vi "Main.vi"() -> ()   [LabVIEW 2017]
uses:
  <vilib>/Platform/TimedLoop/XDataNode/timing_clust.ctl
  <vilib>/Platform/TimedLoop/XDataNode/nitl_modes.ctl
  <vilib>/Platform/TimedLoop/XDataNode/wakeup.ctl
  <vilib>/Analysis/Matrix/Datatypes/RealMatrix.ctl
  <vilib>/Analysis/baseanly.llb/A x Vector.vi
  <vilib>/Analysis/baseanly.llb/Real A x B.vi
  <vilib>/Analysis/_algsub.llb/Real Vector Norm.vi
  <vilib>/Analysis/baseanly.llb/Outer Product.vi
  <vilib>/Analysis/baseanly.llb/Real Outer Product.vi
  <vilib>/robotics/Kinematics/Create Lie Group Matrix.vi
  <vilib>/Analysis/7linalg.llb/Create Special Matrix.vi
  <vilib>/Analysis/7linalg.llb/Create Special Real Matrix.vi
  <vilib>/Analysis/Matrix/Numeric/Multiply/Multiply.vi
  <vilib>/Analysis/Matrix/Numeric/Multiply/Multiply - RM,R.vi
  <vilib>/Analysis/Matrix/Numeric/Multiply/Multiply - R,RM.vi
  <vilib>/Analysis/Matrix/Numeric/Add/Add.vi
  <vilib>/Analysis/Matrix/Numeric/Add/Add - RM,RM.vi
  <vilib>/platform/TimedLoop/XDataNode/XDataNode.xnode
  <vilib>/robotics/Kinematics/NI_Kinematics.lvlib
  <vilib>/Analysis/NI_AALBase.lvlib
  <vilib>/Platform/TimedLoop/XDataNode/XDNodeRunTimeDep.lvlib
  <vilib>/Native 3D Graph/xcontrol/3DPC_SurfacePlot.xctl
  <vilib>/Analysis/Matrix/NI_Matrix.lvlib
  <vilib>/Analysis/NI_AALPro.lvlib
  <vilib>/Native 3D Graph/classes/Base Datatype.lvclass
panel:
  out "W-L":dbl=9.959
  out "break":bool=TRUE
  out "state":dbl[](array[numeric])=[1.0, 0.5, 0.5]
  in  "rom":dbl=0.5
  out "target":dbl[](array[numeric])=[inf, inf, inf] format="%#_15g"
  out "chromosome":dbl[](array[numeric])=[0.20251449555250356, 0.8674619116743827, 0.35840498316248204, 0.9462828018798735, 0.6979927649497852, 0.5023536487970717]
  in  "inertia":dbl=1.0
  out "torque":dbl[](array[numeric])
  in  "radius":dbl=1.0
  in  "damping":dbl=0.5
  out "beta2":dbl=0.7460127831658564
  out "v30":dbl[](array[numeric])=[0.5877852522924729, -0.33935797363675174, -0.7344008870614411]
  out "v10":dbl[](array[numeric])=[0.0, 0.6787159472735029, -0.7344008870614411]
  out "v20":dbl[](array[numeric])=[-0.5877852522924731, -0.3393579736367513, -0.7344008870614411]
  out "dt":dbl=0.001
  in  "period":i64=1
  out "v2":dbl[](array[numeric])=[-0.5877852522924731, -0.3393579736367513, -0.7344008870614411]
  out "v1":dbl[](array[numeric])=[0.0, 0.6787159472735029, -0.7344008870614411]
  out "v3":dbl[](array[numeric])=[0.5877852522924729, -0.33935797363675174, -0.7344008870614411]
  out "theta":dbl[](array[numeric]) format="%#_15g"
  in  "stop":bool
  out "beta1":dbl=0.9553166181245093
  out "gamma2":dbl=1.2566370614359172
  out "gamma1":dbl=1.5707963267948966
  out "alpha2":dbl=1.5707963267948966
  out "alpha1":dbl=1.5707963267948966
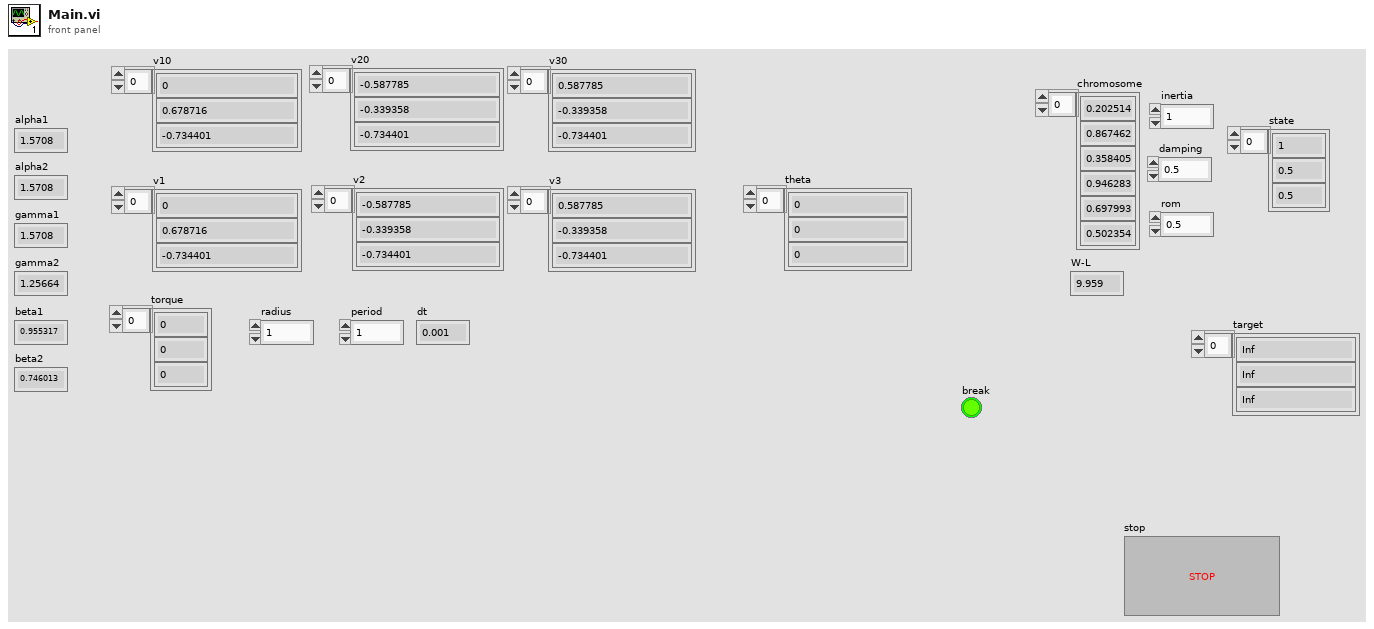
[diagram p1: front panel]
types:
  T1 = typedef "XDNodeRunTimeDep.lvlib/timing_clust.ctl" = cluster{"Expected End [f-1]":u64, "Actual End [f-1]":u64, "Finished Late? [f-1]":bool, "Expected End [i-1]":u64, "Actual End [i-1]":u64, "Finished Late? [i-1]":bool, "Expected Start [i]":u64, "Actual Start [i]":u64, "Expected Start [f]":u64, "Actual Start [f]":u64, "Source Name":string, "Structure Name":string, "Period":i64, "Deadline":i64, "Offset":i64, "Start":i64, "Priority":i32, "Timeout":i32, "Mode":T2, "Wakeup Reason":T3, "Error":errorcluster, "Source Type":string, "Secondary Source Type":string, "Global End Time":u64, "Global Start Time":u64, "Frame Duration":u64, "Iteration Duration":u64, "Assigned CPU":i32, "I/O Scan Engine Mode":u32}
  T2 = typedef "XDNodeRunTimeDep.lvlib/nitl_modes.ctl" = enum32{"No Change", "Process missed periods, maintain original phase", "Discard missed periods, maintain original phase", "Process missed periods, ignore original phase", "Discard missed periods, ignore original phase"}
  T3 = typedef "XDNodeRunTimeDep.lvlib/wakeup.ctl" = enum32{"Normal", "Aborted", "Asynchronous wakeup", "Timing source error", "Timed loop error", "Timeout"}
  T4 = typedef "NI_Matrix.lvlib/RealMatrix.ctl" = dbl[][]
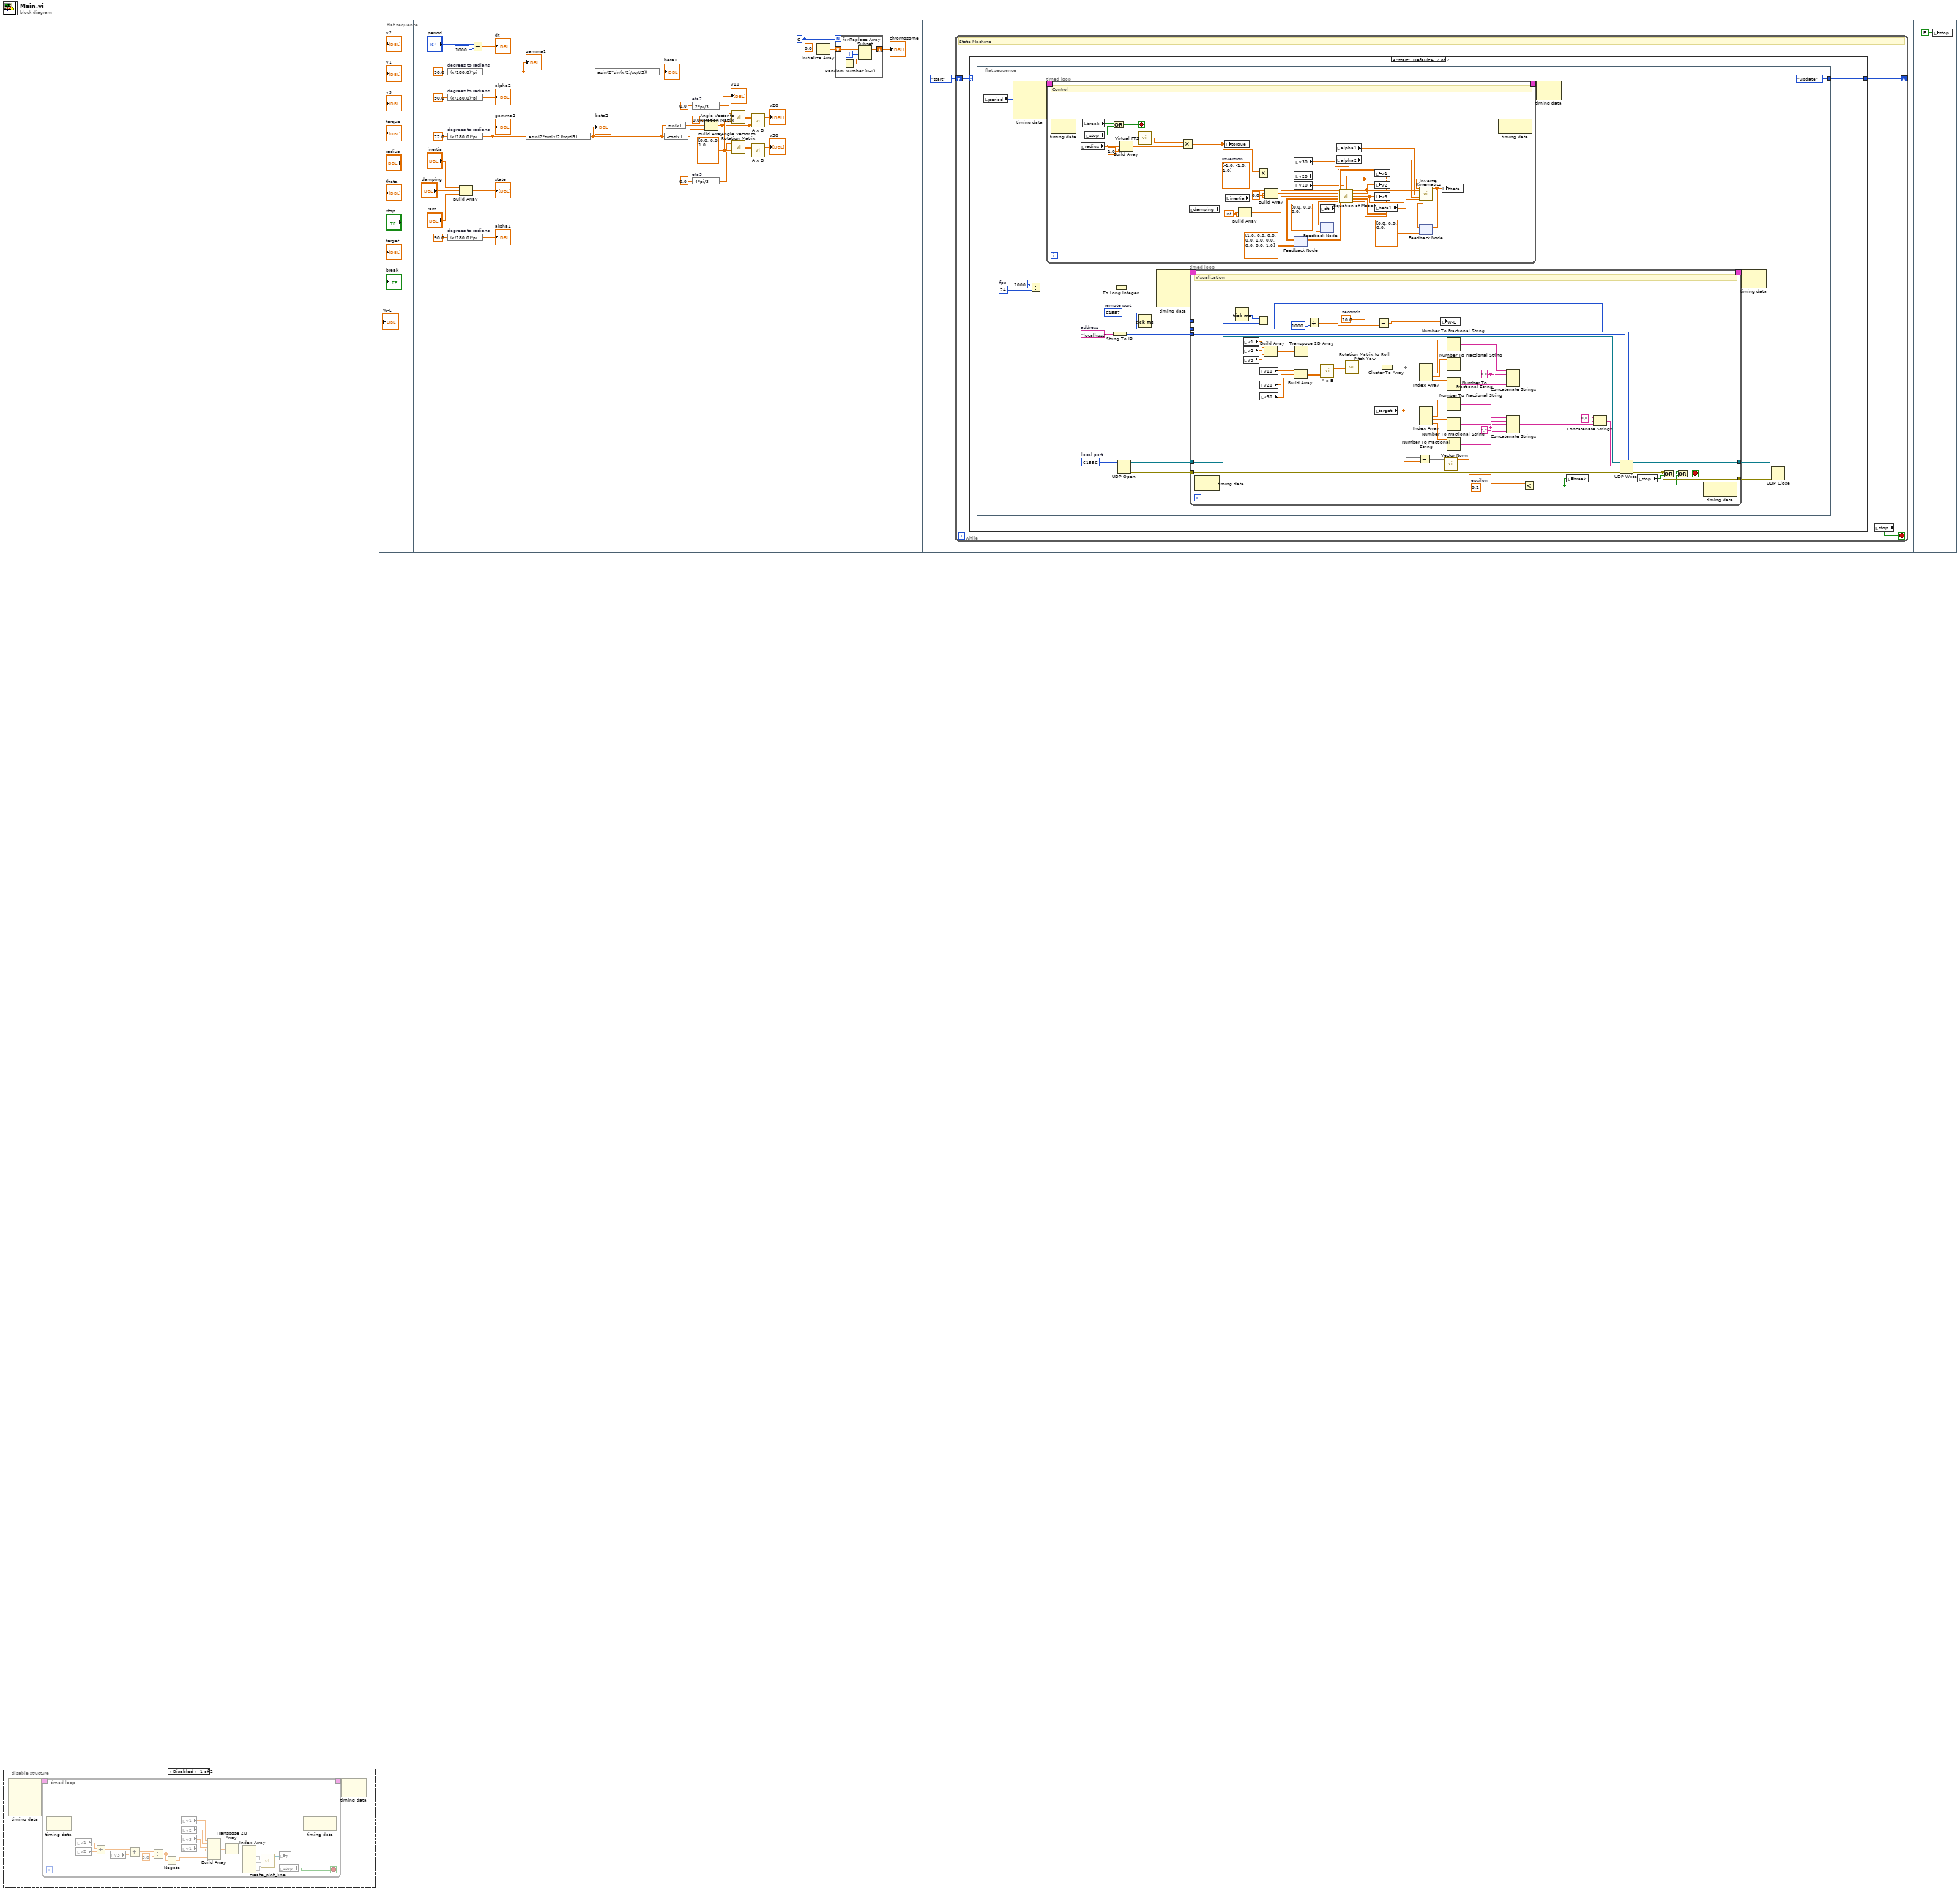
[diagram p0: block diagram]
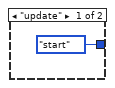
[diagram p3: hidden frame]
diagram:
  n1 = disable-structure shown="Disabled" {
    frame Disabled {
      n2 = node-c288() -> (w2:T1)  [unwired: 4 in]
      n3 = timed-loop {
        timing: w2 -> [_]
        timing-out: [_] -> w1
        stop <- w3 stop-if-true
        n4 = node-c288() -> ()  [unwired: 1 in, 1 out]
        n5 = local read "v1"() -> (w12:dbl[])
        n6 = local read "v2"() -> (w11:dbl[])
        n7 = Add(x=w12, y=w11) -> (x+y=w10:dbl[])
        n8 = local read "v3"() -> (w9:dbl[])
        n9 = Add(x=w10, y=w9) -> (x+y=w8:dbl[])
        n10 = Divide(x=w8, y=3.0) -> (x/y=w6:dbl[])
        n11 = Negate(x=w6) -> (-x=w5:dbl[])
        n12 = local read "v1"() -> (w20:dbl[])
        n13 = local read "v2"() -> (w19:dbl[])
        n14 = local read "v3"() -> (w18:dbl[])
        n15 = local read "v1"() -> (w17:dbl[])
        n16 = Build Array(w20, w19, w18, w17, w6, w5) -> (w16:dbl[][])
        n17 = Transpose 2D Array(2D array=w16) -> (transposed array=w15:dbl[][])
        n18 = Index Array(array=w15) -> (element #1=w14:dbl[], element #2=w13:dbl[], element #3=w4:dbl[])  [unwired: 6 in]
        n19 = call <vilib>:"create_plot_line.vi"("z vector"=w4, "y vector"=w13, "x vector"=w14) -> ("plots out"=w21:refnum<class "Base Datatype.lvclass">[])  [unwired: 2 in, 6 out]
        n20 = local write item#-1(w21) -> ()
        n21 = local read "stop"() -> (w3:bool)
        n22 = node-c288() -> ()  [unwired: 1 in, 1 out]
      }
      n23 = node-c288(w1) -> ()  [unwired: 1 out]
    }
    frame Enabled {
    }
  }
  n24 = flat-sequence {
    frame #0 {
    }
    frame #1 {
      w52 = dbl[] [0.0, 0.0, 1.0] ("vector")
      # "Kinematics Variables"
      n25 = expression code="(x/180.0)*pi" "degrees to radians"(90.0 ("gamma1")) -> (w36:dbl)
      "gamma1" <- w36
      n26 = expression code="(x/180.0)*pi" "degrees to radians"(90.0 ("alpha2")) -> (→"alpha2":dbl)
      n27 = expression code="(x/180.0)*pi" "degrees to radians"(72.0 ("gamma2")) -> (w34:dbl)
      "gamma2" <- w34
      n28 = expression code="(x/180.0)*pi" "degrees to radians"(90.0 ("alpha1")) -> (→"alpha1":dbl)
      n29 = Build Array("inertia", "damping", "rom") -> (→"state":dbl[])
      n30 = Divide(x="period", y=i64 1000) -> (x/y=→"dt":dbl)
      n31 = expression code="asin(2*sin(x/2)/sqrt(3))"(w34) -> (w30:dbl)
      "beta2" <- w30
      n32 = expression code="asin(2*sin(x/2)/sqrt(3))"(w36) -> (→"beta1":dbl)
      n33 = expression code="-cos(x)"(w30) -> (w53:dbl)
      n34 = expression code="sin(x)"(w30) -> (w54:dbl)
      n35 = expression code="2*pi/3" "eta2"(0.0) -> (w51:dbl)
      n36 = expression code="4*pi/3" "eta3"(0.0) -> (w50:dbl)
      n37 = Build Array(0.0 ("element"), w54, w53) -> (w45:dbl[])
      "v10" <- w45
      n38 = call <vilib>:"Angle Vector to Rotation Matrix.vi"("vector"=w52, "angle"=w51) -> ("rotation matrix"=w49:T4)
      n39 = call <vilib>:"Angle Vector to Rotation Matrix.vi"("vector"=w52, "angle"=w50) -> ("rotation matrix"=w48:T4)
      n40 = call-poly <vilib>:"A x B.vi"("Vector"=w45, "A"=w49) -> ("A x Vector"=→"v20":dbl[])  [unwired: 1 out]
      n41 = call-poly <vilib>:"A x B.vi"("Vector"=w45, "A"=w48) -> ("A x Vector"=→"v30":dbl[])  [unwired: 1 out]
    }
    frame #2 {
      w57 = 6
      n42 = Initialize Array(0.0 ("element"), w57) -> (w59:dbl[])
      n43 = for {
        N: w57 -> [_]
        shift-right: [w60] -> w56
        shift-left: w59 -> [w63]
        i -> [w62]
        n44 = Random Number (0-1)() -> (number: 0 to 1=w61:dbl)
        n45 = Replace Array Subset(array=w63, new element=w61, index=w62) -> (w60:dbl[])
      }
      "chromosome" <- w56
    }
    frame #3 {
      # "FK/IK"
      n46 = while {
        shift-right: [w66] -> _
        shift-left: enum16{"update", "start"}."start" -> [w65]
        stop <- w67 stop-if-true
        # "State Machine"
        n47 = case shown="\"start\", Default" w65 {
          tunnel: [enum16{"update", "start"}."start" w69] -> w66
          frame "update" {
          }
          frame "start", Default {
            n48 = flat-sequence {
              tunnel: [enum16{"update", "start"}."update"] -> w69
              frame #0 {
                w76 = 24  # fps
                w78 = "localhost"  # address
                w80 = u16 61557  # remote port
                w83 = u16 61556  # local port
                n49 = local read "period"() -> (w77:i64)
                n50 = node-c288(w77) -> (w87:T1)  [unwired: 3 in]
                n51 = Divide(x=1000, y=w76) -> (x/y=w74:dbl)
                n52 = timed-loop "Timed Loop" {
                  timing: w87 -> [_]
                  timing-out: [_] -> w86
                  stop <- w145 stop-if-true
                  w149 = inf
                  w148 = 0.0 ("element")
                  w165 = dbl[] [-1.0, -1.0, 1.0]  # inversion
                  # "Control"
                  n53 = node-c288() -> ()  [unwired: 1 in, 1 out]
                  n54 = local read "radius"() -> (w162:dbl)
                  n55 = local read "break"() -> (w147:bool)
                  n56 = local read "stop"() -> (w146:bool)
                  n57 = Or(x=w147, y=w146) -> (x .or. y?=w145:bool)
                  n58 = Build Array(w162, w162, 1.0 ("element")) -> (w159:dbl[])
                  n59 = call "Virtual FTS.vi"() -> ("value"=w160:dbl[])
                  n60 = Multiply(x=w160, y=w159) -> (x*y=w158:dbl[])
                  n61 = local read "damping"() -> (w151:dbl)
                  n62 = local write "torque"(w158) -> ()
                  n63 = local read "inertia"() -> (w153:dbl)
                  n64 = Build Array(w151, w149, w149) -> (w150:dbl[])
                  n65 = Multiply(x=w158, y=w165) -> (x*y=w166:dbl[])
                  n66 = Build Array(w153, w148, w148) -> (w152:dbl[])
                  n67 = feedback #1(T4 [[1.0, 0.0, 0.0], [0.0, 1.0, 0.0], [0.0, 0.0, 1.0]] ("R'")) -> (w155:T4)
                  n68 = local read "v30"() -> (w167:dbl[])
                  n69 = local read "v20"() -> (w168:dbl[])
                  n70 = local read "v10"() -> (w169:dbl[])
                  n71 = local read "dt"() -> (w157:dbl)
                  n72 = feedback #2(dbl[] [0.0, 0.0, 0.0] ("flow'")) -> (w156:dbl[])
                  n73 = local read "alpha1"() -> (w176:dbl)
                  n74 = local read "alpha2"() -> (w177:dbl)
                  n75 = call "Equation of Motion.vi"("torque"=w166, "v10"=w169, "v20"=w168, "v30"=w167, "inertia"=w152, "damping"=w150, "R"=w155, "omega"=w156, "dt"=w157) -> ("v1d"=w174:dbl[], "v2d"=w173:dbl[], "v3d"=w172:dbl[], "R'"=w171:T4, "omega'"=w164:dbl[])  [unwired: 2 in]
                  n76 = feedback-in #1(w171) -> ()
                  n77 = feedback-in #2(w164) -> ()
                  n78 = local write "v1"(w174) -> ()
                  n79 = local write "v2"(w173) -> ()
                  n80 = local write "v3"(w172) -> ()
                  n81 = local read "beta1"() -> (w178:dbl)
                  n82 = feedback #3(dbl[] [0.0, 0.0, 0.0] ("theta0")) -> (w179:dbl[])
                  n83 = call "Inverse Kinematics.vi"("v1"=w174, "v2"=w173, "v3"=w172, "alpha1"=w176, "alpha2"=w177, "beta1"=w178, "theta"=w179) -> ("theta'"=w175:dbl[])  [unwired: 12 in]
                  n84 = feedback-in #3(w175) -> ()
                  n85 = local write "theta"(w175) -> ()
                  n86 = node-c288() -> ()  [unwired: 1 in, 1 out]
                }
                n87 = String To IP(1:w78) -> (0:w79:u32)
                n88 = To Long Integer(number=w74) -> (32bit integer=w73:i32)
                n89 = UDP Open(11:w83) -> (port=w82:refnum<k16>, 0:w72:errorcluster)  [unwired: 4 in, 1 out]
                n90 = Tick Count (ms)() -> (millisecond timer value=w70:u32)
                n91 = node-c288(w73) -> (w85:T1)  [unwired: 3 in]
                n92 = timed-loop "Timed Loop" {
                  timing: w85 -> [_]
                  timing-out: [_] -> w84
                  tunnel: w82 -> [w138]
                  tunnel: [w137] -> w81
                  tunnel: w80 -> [w129]
                  tunnel: w79 -> [w128]
                  tunnel: w72 -> [w116]
                  tunnel: [w114] -> w71
                  tunnel: w70 -> [w94]
                  stop <- w93 stop-if-true
                  w89 = 10.0  # seconds
                  w98 = 0.1  # epsilon
                  w127 = "," ("string")
                  w130 = "," ("string")
                  # "Visualization"
                  n93 = node-c288() -> ()  [unwired: 1 in, 1 out]
                  n94 = Tick Count (ms)() -> (millisecond timer value=w95:u32)
                  n95 = local read "v1"() -> (w113:dbl[])
                  n96 = local read "v2"() -> (w112:dbl[])
                  n97 = local read "v3"() -> (w111:dbl[])
                  n98 = Subtract(x=w95, y=w94) -> (x-y=w92:u32)
                  n99 = local read "v10"() -> (w108:dbl[])
                  n100 = local read "v20"() -> (w109:dbl[])
                  n101 = local read "v30"() -> (w110:dbl[])
                  n102 = Build Array(w113, w112, w111) -> (w107:dbl[][])
                  n103 = Build Array(w108, w109, w110) -> (w105:dbl[][])
                  n104 = Transpose 2D Array(2D array=w107) -> (transposed array=w106:dbl[][])
                  n105 = Divide(x=w92, y=u32 1000) -> (x/y=w90:dbl)
                  n106 = call-poly <vilib>:"A x B.vi"("B"=w105, "A"=w106) -> ("A x B"=w104:T4)  [unwired: 1 out]
                  n107 = call <vilib>:"Rotation Matrix to Roll Pitch Yaw.vi"("rotation matrix"=w104) -> ("angles"=w103:cluster{"roll":dbl, "pitch":dbl, "yaw":dbl})
                  n108 = local read "target"() -> (w101:dbl[])
                  n109 = Subtract(x=w89, y=w90) -> (x-y=w88:dbl)
                  n110 = Cluster To Array(cluster=w103) -> (array=w102:dbl[])
                  n111 = Subtract(x=w102, y=w101) -> (x-y=w100:dbl[])
                  n112 = Index Array(array=w102) -> (element #1=w136:dbl, element #2=w135:dbl, element #3=w134:dbl)  [unwired: 3 in]
                  n113 = Index Array(array=w101) -> (element #1=w123:dbl, element #2=w122:dbl, element #3=w121:dbl)  [unwired: 3 in]
                  n114 = local write "W-L"(w88) -> ()
                  n115 = call-poly <vilib>:"Vector Norm.vi"("Input Vector"=w100) -> ("norm"=w99:dbl)  [unwired: 9 in, 1 out]
                  n116 = Number To Fractional String(number=w136) -> (F-format string=w133:string)  [unwired: 3 in]
                  n117 = Number To Fractional String(number=w135) -> (F-format string=w132:string)  [unwired: 3 in]
                  n118 = Number To Fractional String(number=w134) -> (F-format string=w131:string)  [unwired: 3 in]
                  n119 = Number To Fractional String(number=w123) -> (F-format string=w124:string)  [unwired: 3 in]
                  n120 = Number To Fractional String(number=w122) -> (F-format string=w125:string)  [unwired: 3 in]
                  n121 = Number To Fractional String(number=w121) -> (F-format string=w126:string)  [unwired: 3 in]
                  n122 = Concatenate Strings(w133, w130, w132, w130, w131) -> (w119:string)
                  n123 = Concatenate Strings(w124, w127, w125, w127, w126) -> (w118:string)
                  n124 = Less?(x=w99, y=w98) -> (x < y?=w96:bool)
                  n125 = local write "break"(w96) -> ()
                  n126 = Concatenate Strings(w119, "," ("string"), w118) -> (w117:string)
                  n127 = UDP Write(address=w128, port or service name=w129, connection ID=w138, data in=w117, 8:w116) -> (error out=w114:errorcluster, 3:w137:refnum<k16>)  [unwired: 1 in]
                  n128 = local read "stop"() -> (w115:bool)
                  n129 = Or(x=w114, y=w115) -> (x .or. y?=w97:bool)
                  n130 = Or(x=w97, y=w96) -> (x .or. y?=w93:bool)
                  n131 = node-c288() -> ()  [unwired: 1 in, 1 out]
                }
                n132 = node-c288(w86) -> ()  [unwired: 1 out]
                n133 = node-c288(w84) -> ()  [unwired: 1 out]
                n134 = UDP Close(connection ID=w81, 8:w71) -> ()  [unwired: 2 out]
              }
              frame #1 {
              }
            }
          }
        }
        n135 = local read "stop"() -> (w67:bool)
      }
    }
    frame #4 {
      n136 = local write "stop"(FALSE ("stop")) -> ()
    }
  }
